vi "SPD.Get Results Folder.vi"(8 "Error In":errorcluster, 10 "Temperature":dbl, 11 "SPD.Stand Ctrl in":T1 {"spdDeviceSession"."hidSPD.Sturtup Values"."HV_bias" format="%#_6p, V"; "spdDeviceSession"."hidSPD.Sturtup Values"."TSet" format="%#_6p, DegC"; "spdDeviceSession"."hidSPD.Controller"."HV_bias" format="%#_6p, V"; "spdDeviceSession"."hidSPD.Controller"."TSet" format="%#_6p, DegC"}) -> (0 "Error Out":errorcluster, 2 "Results path":path, 3 "SPD.Stand Ctrl out":T1 {"spdDeviceSession"."hidSPD.Sturtup Values"."HV_bias" format="%#_6p, V"; "spdDeviceSession"."hidSPD.Sturtup Values"."TSet" format="%#_6p, DegC"; "spdDeviceSession"."hidSPD.Controller"."HV_bias" format="%#_6p, V"; "spdDeviceSession"."hidSPD.Controller"."TSet" format="%#_6p, DegC"})   [LabVIEW 2018]
uses:
  typedefs/SPD.Stand Ctrl.ctl
  Instruments/SPD HID Interface/hidSPDLibForLabView/LibVIs/hidSPD Controls/hidSPD Device Session.ctl
  Instruments/SPD HID Interface/hidSPDLibForLabView/LibVIs/hidSPD Controls/hidSPD Controller.ctl
  Instruments/SPD HID Interface/hidSPDLibForLabView/LibVIs/hidSPD Controls/hidSPD SPD Type.ctl
  Instruments/KC705 DevBoard/typedefs/DevB.Session.ctl
  Instruments/KeySight 53230A/typedefs/FreqC.Session.ctl
  Instruments/KeySight 8164B/KeySight 8164B LAN InstrLib/typedefs/KeySight 8164B control.ctl
  Instruments/LeCroy SDA830/typedefs/LeCroy.Session.ctl
  typedefs/SPD.Events.ctl
  ConfigFile/SPD.Config File ctrl.ctl
  <vilib>/Utility/config.llb/Config Data RefNum.ctl
  typedefs/SPD.Meas Result.ctl
  typedefs/SPD.Queues.ctl
  typedefs/SPD.Stand state.ctl
  <vilib>/Utility/sysdir.llb/System Directory Type.ctl
  Instruments/KeySight 8164B/KeySight 8164B LAN InstrLib.lvlib
  <vilib>/Utility/config.llb/NI_LVConfig.lvlib
  Instruments/SPD HID Interface/hidSPDLibForLabView/hidSPDLibForLabView.lvlib
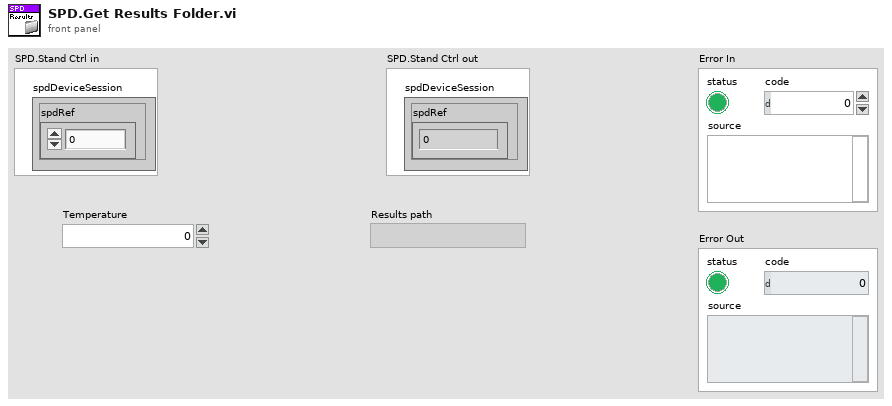
[diagram p1: front panel]
types:
  T1 = typedef "SPD.Stand Ctrl.ctl" = cluster{"spdDeviceSession":T2, "DevBSession":T5, "FreqCSession":T6, "8164BSession":T7, "LeCroySession":T8, "Events":T9, "configFile":T10, "SPD.Result":T12, "SPD.Queues":T13, "Console":refnum<vi>}
  T2 = typedef "hidSPDLibForLabView.lvlib/hidSPD Device Session.ctl" = cluster{"spdRef":u64, "connected":bool, "spdName":string, "hidSPD.Controller":T3, "hidSPD.Sturtup Values":T3, "SPD Type":T4}
  T3 = typedef "hidSPDLibForLabView.lvlib/hidSPD Controller.ctl" = cluster{"TSet":sgl, "HV_bias":sgl, "DDS_stb_code":u16}
  T4 = typedef "hidSPDLibForLabView.lvlib/hidSPD SPD Type.ctl" = enum16{"Free Run", "Strobe"}
  T5 = typedef "DevB.Session.ctl" = cluster{"DevBRef":refnum<visa-resource-name>, "connected":bool}
  T6 = typedef "FreqC.Session.ctl" = cluster{"FreqCRef":refnum<visa-resource-name>, "timeout":dbl, "Gate":dbl, "connected":bool}
  T7 = typedef "KeySight 8164B LAN InstrLib.lvlib/KeySight 8164B control.ctl" = cluster{"Connection ID":refnum<k5>, "Connected":bool, "Info":string, "Slots Info":string[]}
  T8 = typedef "LeCroy.Session.ctl" = cluster{"LeCroySession":refnum<visa-resource-name>, "connected":bool}
  T9 = typedef "SPD.Events.ctl" = cluster{"DCRTest":refnum<user-event>, "Stop":refnum<user-event>}
  T10 = typedef "SPD.Config File ctrl.ctl" = cluster{"configFile ref":T11, "configFile path":path, "equipmentFile ref":T11}
  T11 = typedef "NI_LVConfig.lvlib/Config Data RefNum.ctl" = refnum<k1>
  T12 = typedef "SPD.Meas Result.ctl" = cluster{"HV_Bias":dbl[][][], "Stb_code":dbl[], "Temprature":dbl[], "Data":dbl[][][][], "DateTime":string}
  T13 = typedef "SPD.Queues.ctl" = cluster{"state queue":refnum<queue>}
  T14 = typedef "System Directory Type.ctl" = i32
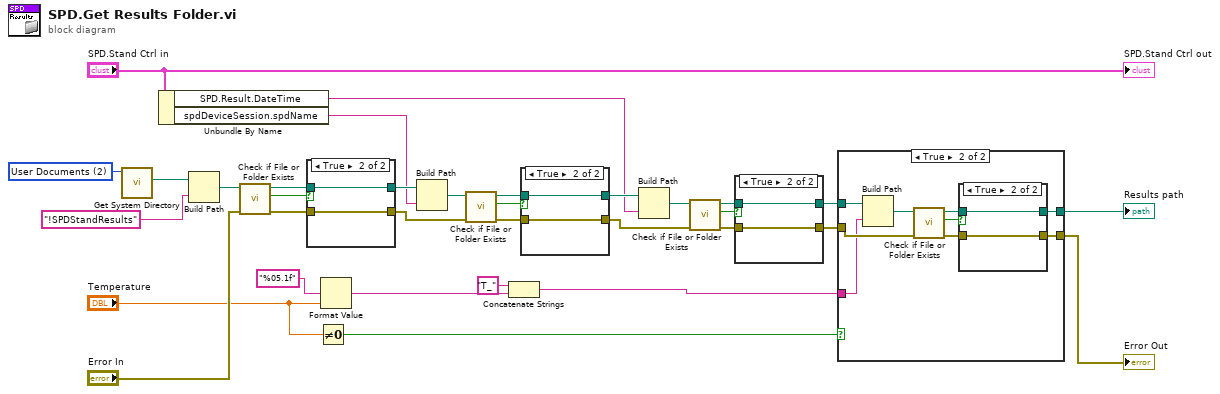
[diagram p0: block diagram]
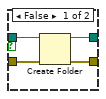
[diagram p3: hidden frame]
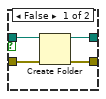
[diagram p4: hidden frame]
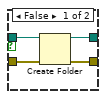
[diagram p5: hidden frame]
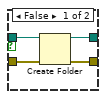
[diagram p6: hidden frame]
diagram:
  w33 = T14 2 items=["User Home"=0, "User Desktop"=1, "User Documents"=2, "User Application Data"=3, "User Preferences"=4, "User Temporary"=5, "Public Documents"=6, "Public Application Data"=7, "Public Preferences"=8, "Public Cache"=13, "System Core Libraries"=9, "System Installed Libraries"=10, "Application Files"=11, "Boot Volume Root"=12] ("system directory type")
  n1 = call <vilib>:"Get System Directory.vi"("system directory type"=w33) -> ("system directory"=w32:path)  [unwired: 10 in]
  n2 = Unbundle By Name("SPD.Stand Ctrl in") -> ("SPD.Result.DateTime"=w16:string, "spdDeviceSession.spdName"=w23:string)
  n3 = Build Path(base path=w32, name or relative path="!SPDStandResults") -> (appended path=w30:path)
  n4 = call <vilib>:"Check if File or Folder Exists.vi"("error in (no error)"="Error In", "path"=w30) -> ("error out"=w26:errorcluster, "file or folder exists?"=w28:bool, "dup path"=w27:path)  [unwired: 7 in]
  n5 = case shown="True" w28 {
    tunnel: w27 -> [w37 w39]
    tunnel: w26 -> [w36 w38]
    tunnel: [w35 w39] -> w25
    tunnel: [w34 w38] -> w21
    frame False {
      n6 = Create Folder(path (use dialog)=w37, error in=w36) -> (created path=w35:path, error out=w34:errorcluster)  [unwired: 1 in, 1 out]
    }
    frame True {
    }
  }
  n7 = Not Equal To 0?(x="Temperature") -> (x != 0?=w3:bool)
  n8 = Format Value(format string="%05.1f", value (0)="Temperature") -> (output string=w5:string)  [unwired: 1 in]
  n9 = Build Path(base path=w25, name or relative path=w23) -> (appended path=w22:path)
  n10 = call <vilib>:"Check if File or Folder Exists.vi"("error in (no error)"=w21, "path"=w22) -> ("error out"=w18:errorcluster, "file or folder exists?"=w19:bool, "dup path"=w20:path)  [unwired: 7 in]
  n11 = Concatenate Strings("T_" ("string"), w5) -> (w2:string)
  n12 = case shown="True" w19 {
    tunnel: w20 -> [w43 w45]
    tunnel: w18 -> [w42 w44]
    tunnel: [w41 w45] -> w17
    tunnel: [w40 w44] -> w14
    frame False {
      n13 = Create Folder(path (use dialog)=w43, error in=w42) -> (created path=w41:path, error out=w40:errorcluster)  [unwired: 1 in, 1 out]
    }
    frame True {
    }
  }
  n14 = Build Path(base path=w17, name or relative path=w16) -> (appended path=w15:path)
  n15 = call <vilib>:"Check if File or Folder Exists.vi"("error in (no error)"=w14, "path"=w15) -> ("error out"=w11:errorcluster, "file or folder exists?"=w12:bool, "dup path"=w13:path)  [unwired: 7 in]
  n16 = case shown="True" w12 {
    tunnel: w13 -> [w49 w51]
    tunnel: w11 -> [w48 w50]
    tunnel: [w47 w51] -> w10
    tunnel: [w46 w50] -> w9
    frame False {
      n17 = Create Folder(path (use dialog)=w49, error in=w48) -> (created path=w47:path, error out=w46:errorcluster)  [unwired: 1 in, 1 out]
    }
    frame True {
    }
  }
  n18 = case shown="True" w3 {
    tunnel: w10 -> [w53 w58]
    tunnel: w9 -> [w52 w57]
    tunnel: [w53 w56] -> w8
    tunnel: [w52 w55] -> w7
    tunnel: w2 -> [_ w54]
    frame False {
    }
    frame True {
      n19 = Build Path(base path=w58, name or relative path=w54) -> (appended path=w59:path)
      n20 = call <vilib>:"Check if File or Folder Exists.vi"("error in (no error)"=w57, "path"=w59) -> ("error out"=w62:errorcluster, "file or folder exists?"=w61:bool, "dup path"=w60:path)  [unwired: 7 in]
      n21 = case shown="True" w61 {
        tunnel: w60 -> [w66 w68]
        tunnel: w62 -> [w65 w67]
        tunnel: [w64 w68] -> w56
        tunnel: [w63 w67] -> w55
        frame False {
          n22 = Create Folder(path (use dialog)=w66, error in=w65) -> (created path=w64:path, error out=w63:errorcluster)  [unwired: 1 in, 1 out]
        }
        frame True {
        }
      }
    }
  }
  "Error Out" <- w7
  "Results path" <- w8
  "SPD.Stand Ctrl out" <- "SPD.Stand Ctrl in"
